vi "Multi Accelerometer Event Example.vi"() -> ()   [LabVIEW 2012, in "Phidget Common.lvlib"]
uses:
  <instrlib>/Phidgets/Phidget Common/Phidget Common.lvlib
  <instrlib>/Phidgets/Phidget Accelerometer/Public/AccelerometerStart.vi
  <instrlib>/Phidgets/Phidget Accelerometer/Public/AccelerometerClose.vi
  <instrlib>/Phidgets/Phidget Accelerometer/Phidget Accelerometer.lvlib
panel:
  out "Timestamp 2":u64
  out "Data 2":dbl[](array[numeric])
  out "Serial Number Return 2":i32
  in  "Device Info 2":T1={"Serial Number"=-1, "Channel"=0, "Port"=0}
  out "Timestamp":u64
  in  "stop":bool
  out "Serial Number Return":i32
  in  "Device Info":T1={"Serial Number"=-1, "Channel"=0, "Port"=0}
  out "Data":dbl[](array[numeric])
  out "error out":errorcluster
  # "Be sure to use this stop button to stop the program.\nIf you use the \"Abort Execution\" button, you will\nneed to use PhidgetResetLibrary.vi or restart Labview \nin order for any Phidgets to work."
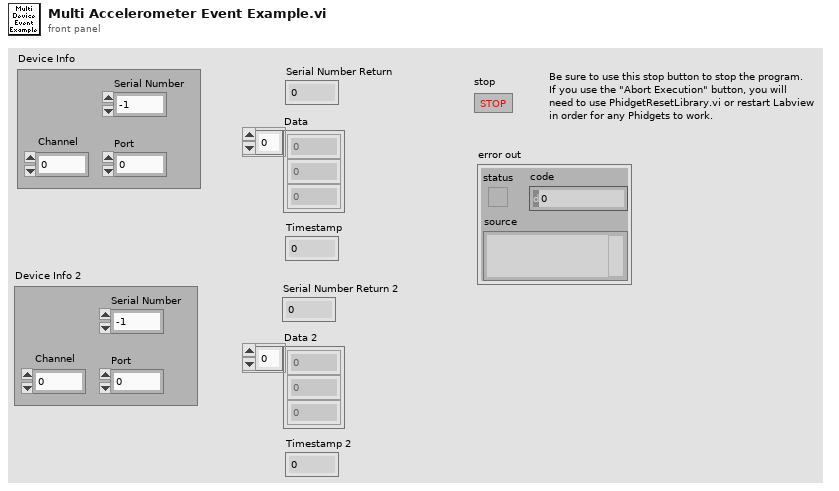
[diagram p1: front panel]
types:
  T1 = cluster{"Serial Number":i32, "Channel":i32, "Port":i32}
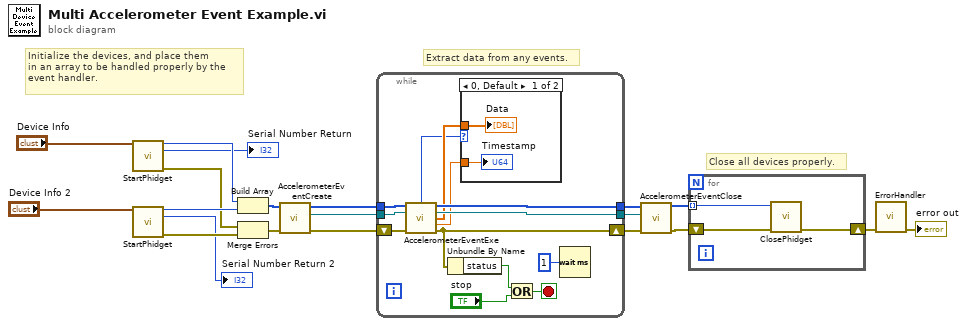
[diagram p0: block diagram]
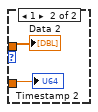
[diagram p2: hidden frame]
diagram:
  # "Close all devices properly."
  # "Extract data from any events."
  # "Initialize the devices, and place them\nin an array to be handled properly by the\nevent handler."
  n1 = call-poly <instrlib>:"StartPhidget.vi"("Device Info"="Device Info") -> ("Phidget ID"=w9:u64, "Serial Number Return"=→"Serial Number Return":i32, "error out"=w4:errorcluster)  [unwired: 11 in, 1 out]
  n2 = call-poly <instrlib>:"StartPhidget.vi"("Device Info"="Device Info 2") -> ("Phidget ID"=w5:u64, "Serial Number Return"=→"Serial Number Return 2":i32, "error out"=w3:errorcluster)  [unwired: 11 in, 1 out]
  n3 = Build Array(w9, w5) -> (w20:u64[])
  n4 = Merge Errors(w4, w3) -> (w11:errorcluster)
  n5 = call <instrlib>:"AccelerometerEventCreate.vi"("error in (no error)"=w11, "Devices In"=w20) -> ("error out"=w13:errorcluster, "Event Registration Refnum"=w18:refnum<event-registration>, "Devices Out"=w19:u64[])  [unwired: 7 in]
  n6 = while {
    tunnel: w19 -> [w33]
    tunnel: w18 -> [w28]
    tunnel: [w32] -> w15
    shift-right: [w27] -> w14
    shift-left: w13 -> [w31]
    tunnel: [w29] -> w7
    stop <- w26 stop-if-true
    n7 = call <instrlib>:"AccelerometerEventExe.vi"("Devices In"=w33, "Event Registration Refnum In"=w28, "error in (no error)"=w31) -> ("Index"=w21:i32, "Devices Out"=w29:u64[], "Event Registration Refnum Out"=w32:refnum<event-registration>, "Accel Data"=w22:dbl[], "Timestamp"=w23:dbl, "error out"=w27:errorcluster)  [unwired: 5 in, 2 out]
    n8 = Unbundle By Name(w27) -> ("status"=w24:bool)
    n9 = case shown="0, Default" w21 {
      tunnel: w23 -> [w35 w36]
      tunnel: w22 -> [w34 w37]
      frame 0, Default {
        "Data" <- w34
        "Timestamp" <- w35
      }
      frame 1 {
        "Data 2" <- w37
        "Timestamp 2" <- w36
      }
    }
    n10 = Or(x=w24, y="stop") -> (x .or. y?=w26:bool)
    n11 = Wait (ms)(milliseconds to wait=u32 1) -> ()  [unwired: 1 out]
  }
  n12 = call <instrlib>:"AccelerometerEventClose.vi"("error in (no error)"=w14, "Event Registration Refnum In"=w15, "Devices In"=w7) -> ("error out"=w10:errorcluster, "Devices Out"=w8:u64[])  [unwired: 7 in]
  n13 = for {
    tunnel: w8 -> [w38] mode=indexing
    shift-right: [w40] -> w17
    shift-left: w10 -> [w39]
    n14 = call-poly <instrlib>:"ClosePhidget.vi"("error in"=w39, "Device In"=w38) -> ("error out"=w40:errorcluster)  [unwired: 9 in]
  }
  n15 = call <instrlib>:"ErrorHandler.vi"("error in"=w17) -> ("error out"=→"error out":errorcluster)  [unwired: 9 in, 1 out]
